vi "19-AddBeacons.vi"(9 "Base Orientation Info in":T2, 10 "Match Info":T3, 11 "Orientation Info in":T2) -> (1 "Base Orientation Info out":T2, 2 "Sensor Match Info":T1)   [LabVIEW 2019, in "19.lvlib"]
uses:
  19.lvlib
  369ab621-13d8-4e94-865d-419521943cf8.vi
  <vilib>/Array/Sort 2D Array - Pop Stack.vi
  <vilib>/Array/Sort 2D Array - Push Stack.vi
  369ab621-13d8-4e94-865d-419521943cf8.vi/b0a630e8-162a-415a-ac74-39e052cc49ad.vi
  369ab621-13d8-4e94-865d-419521943cf8.vi/57529e2f-0bbf-4816-95bf-97653d082a1e.vi
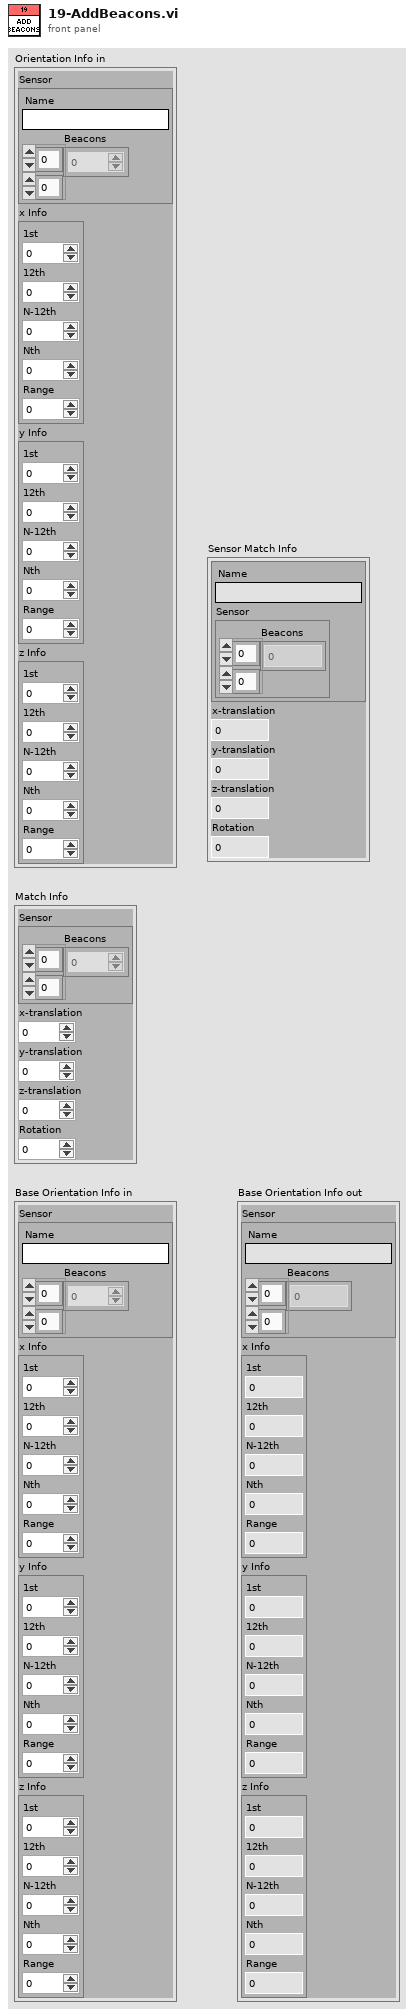
[diagram p1: front panel]
types:
  T1 = cluster{cluster{"Name":string, "Sensor":cluster{"Beacons":i32[][]}}, "x-translation":i32, "y-translation":i32, "z-translation":i32, "Rotation":i32}
  T2 = cluster{"Sensor":cluster{"Name":string, "Beacons":i32[][]}, "x Info":cluster{"1st":i32, "12th":i32, "N-12th":i32, "Nth":i32, "Range":i32}, "y Info":cluster{"1st":i32, "12th":i32, "N-12th":i32, "Nth":i32, "Range":i32}, "z Info":cluster{"1st":i32, "12th":i32, "N-12th":i32, "Nth":i32, "Range":i32}}
  T3 = cluster{"Sensor":cluster{"Beacons":i32[][]}, "x-translation":i32, "y-translation":i32, "z-translation":i32, "Rotation":i32}
  T4 = cluster{"Name":string, "Sensor":cluster{"Beacons":i32[][]}}
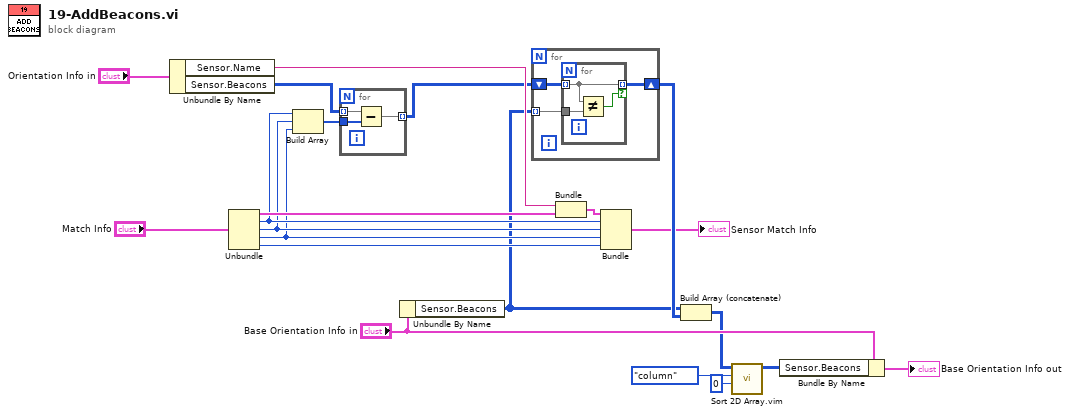
[diagram p0: block diagram]
diagram:
  n1 = Unbundle By Name("Orientation Info in") -> ("Sensor.Name"=w16:string, "Sensor.Beacons"=w7:i32[][])
  n2 = Unbundle("Match Info") -> ("Sensor"=w17:cluster{"Beacons":i32[][]}, "x-translation"=w11:i32, "y-translation"=w9:i32, "z-translation"=w8:i32, "Rotation"=w13:i32)
  n3 = Build Array(w11, w9, w8) -> (w10:i32[])
  n4 = for {
    tunnel: w7 -> [w24] mode=indexing
    tunnel: w10 -> [w23]
    tunnel: [w22] -> w6 mode=indexing
    n5 = Subtract(x=w24, y=w23) -> (x-y=w22:i32[])
  }
  n6 = Unbundle By Name("Base Orientation Info in") -> ("Sensor.Beacons"=w1:i32[][])
  n7 = for {
    shift-right: [w25] -> w21
    shift-left: w6 -> [w27]
    tunnel: w1 -> [w26] mode=indexing
    n8 = for {
      tunnel: w27 -> [w29] mode=indexing
      tunnel: [w29] -> w25 mode=indexing if=w28
      tunnel: w26 -> [w30]
      n9 = Not Equal?(x=w29, y=w30) -> (x != y?=w28:bool)
    }
  }
  n10 = Bundle("Name"=w16, "Sensor"=w17) -> (w14:T4)  [unwired: 1 in]
  n11 = Bundle(w14, "x-translation"=w11, "y-translation"=w9, "z-translation"=w8, "Rotation"=w13) -> (→"Sensor Match Info":T1)  [unwired: 1 in]
  n12 = Build Array (concatenate)(w1, w21) -> (w4:i32[][])
  n13 = call "Sort 2D Array.vim"("index"=0, "dimension to index (column)"=enum16{"column", "row"}."column", "2D array"=w4) -> ("sorted 2D array"=w5:i32[][])  [unwired: 7 in, 1 out]
  n14 = Bundle By Name(cluster="Base Orientation Info in", "Sensor.Beacons"=w5) -> (→"Base Orientation Info out":T2)
